vi "PathPlanner_GeomUtil_DoubleLerp.vi"(9 "T":dbl, 10 "EndVal":dbl, 11 "StartVal":dbl) -> (3 "Lerp":dbl)   [LabVIEW 2019, in "PathPlanner24.lvlib"]
doc: "Interpolate between two doubles\n\nInputs: \n - startVal - double - Start value\n - endVal - double - End value\n - t - double - Interpolation factor (0.0-1.0)\n\nOutputs:\n - Lerp - double - Interpolated value"
uses:
  PathPlanner24.lvlib
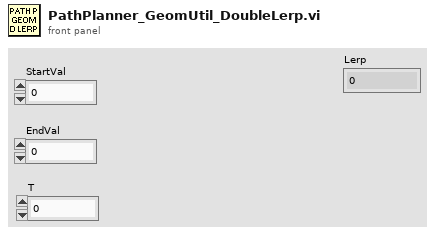
[diagram p1: front panel]
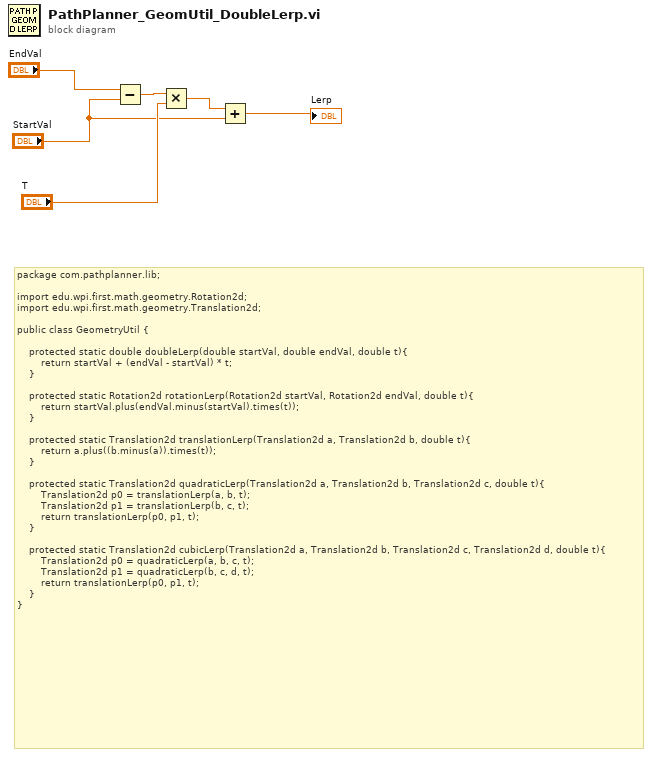
[diagram p0: block diagram]
diagram:
  # "package com.pathplanner.lib;\n\nimport edu.wpi.first.math.geometry.Rotation2d;\nimport edu.wpi.first.math.geometry.Translation2d;\n\npublic class GeometryUtil {\n\n    protected static double doubleLerp(double startVal, double endVal, double t){\n        return startVal + (endVal - startVal) * t;\n    }\n\n    protected static Rotation2d rotationLerp(Rotation2d startVal, Rotation2d endVal, double t){\n        return startVal.plus(endVal.minus(startVal).times(t));\n    }\n\n    protected static Translation2d translationLerp(Translation2d a, Translation2d b, double t){\n        return a.plus((b.minus(a)).times(t));\n    }\n\n    protected static Translation2d quadraticLerp(Translation2d a, Translation2d b, Translation2d c, double t){\n        Translation2d p0 = translationLerp(a, b, t);\n        Translation2d p1 = translationLerp(b, c, t);\n        return translationLerp(p0, p1, t);\n    }\n\n    protected static Translation2d cubicLerp(Translation2d a, Translation2d b, Translation2d c, Translation2d d, double t){\n        Translation2d p0 = quadraticLerp(a, b, c, t);\n        Translation2d p1 = quadraticLerp(b, c, d, t);\n        return translationLerp(p0, p1, t);\n    }\n}"
  n1 = Subtract(x="EndVal", y="StartVal") -> (x-y=w4:dbl)
  n2 = Multiply(x=w4, y="T") -> (x*y=w3:dbl)
  n3 = Add(x=w3, y="StartVal") -> (x+y=→"Lerp":dbl)
